vi "TCP.IP Server for Ripple Detection - edited for data 2.vi"() -> ()   [LabVIEW 2021]
doc: "Demonstrates how to set up a basic TCP connection, send data to the specified port once a connection has been established, and terminate the connection once the data has been sent. This VI is designed to stop if the TCP connection is terminated. The data sent in this example is an array of random numbers."
panel:
  out "error out":errorcluster
  in  "error in (no error)":errorcluster
  out "Numeric 3":dbl
  out "Waveform Graph 10":dynamicdata(graph)
  in  "loop 1":i32
  in  "Client Closed":string="The client VI closed the connection."
  in  "Stop":bool
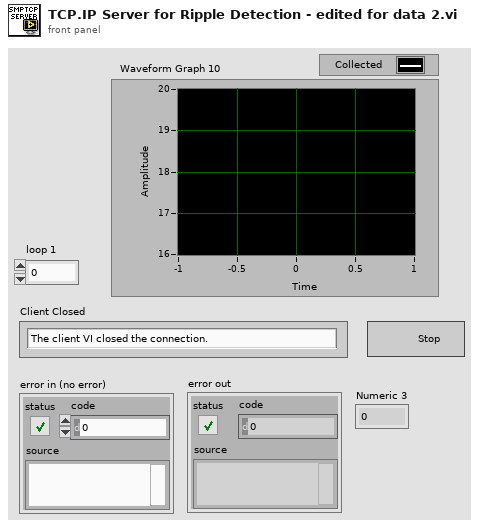
[diagram p1: front panel]
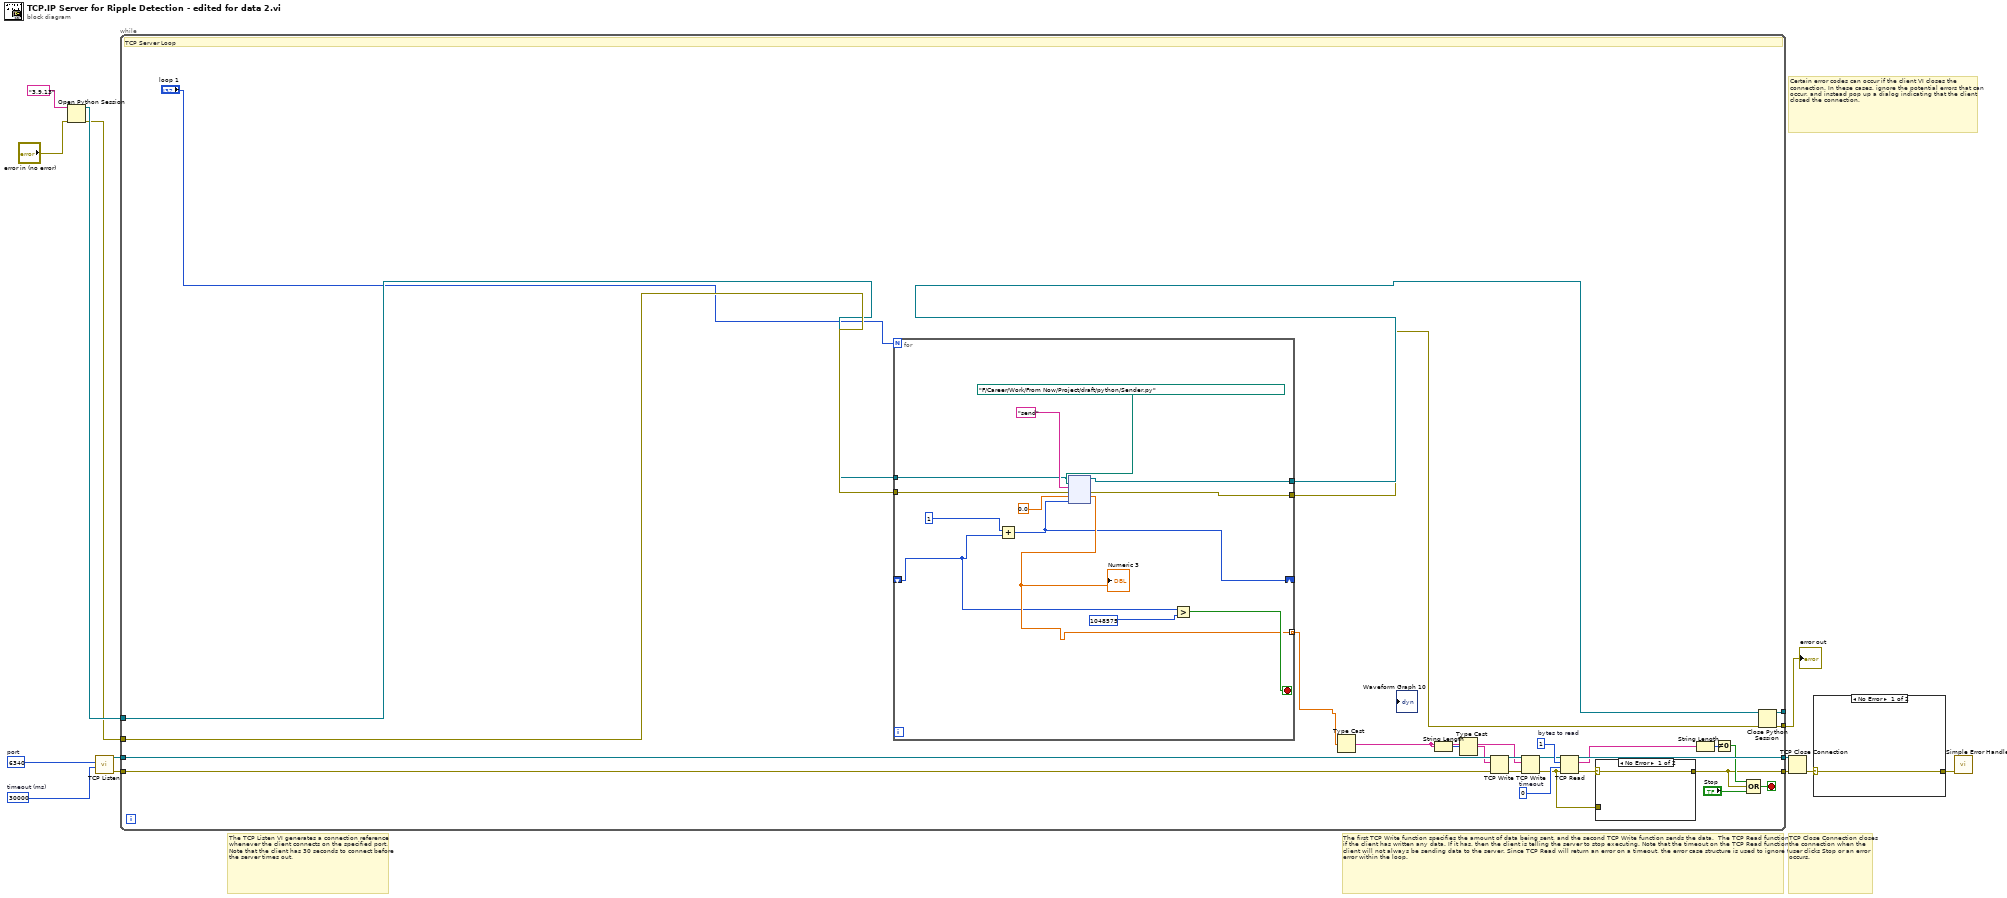
[diagram p0: block diagram]
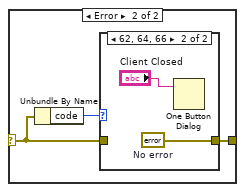
[diagram p2: hidden frame]
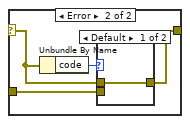
[diagram p4: hidden frame]
diagram:
  w8 = u16 6340  # port
  w9 = 30000  # timeout (ms)
  # "TCP Close Connection closes the connection when the user clicks Stop or an error occurs."
  # "The TCP Listen VI generates a connection reference whenever the client connects on the specified port. Note that the client has 30 seconds to connect before the server times out."
  # "Certain error codes can occur if the client VI closes the connection. In these cases, ignore the potential errors that can occur, and instead pop up a dialog indicating that the client closed the connection."
  # "The first TCP Write function specifies the amount of data being sent, and the second TCP Write function sends the data.  The TCP Read function checks to see if the client has written any data. If it has, then the client is telling the server to stop executing. Note that the timeout on the TCP Read function is '0', as the client will not always be sending data to the server. Since TCP Read will return an error on a timeout, the error case structure is used to ignore the timeout error within the loop."
  n1 = Open Python Session(python version="3.9.13" ("Python version"), 3:"error in (no error)") -> (session out=w6:refnum<k35>, error out=w5:errorcluster)  [unwired: 1 in]
  n2 = call <vilib>:"TCP Listen.vi"("timeout ms (wait forever: -1)"=w9, "port"=w8) -> ("error out"=w10:errorcluster, "connection ID"=w11:refnum<k5>)  [unwired: 5 in, 3 out]
  n3 = while {
    tunnel: [w23] -> w14
    tunnel: [w29] -> w15
    tunnel: w11 -> [w40]
    tunnel: w10 -> [w33]
    tunnel: w6 -> [w18]
    tunnel: w5 -> [w19]
    tunnel: [w21] -> w4
    tunnel: [w20] -> w3
    stop <- w34 stop-if-true
    w28 = 0  # timeout
    w31 = 1  # bytes to read
    # "TCP Server Loop"
    n4 = for {
      N: "loop 1" -> [_]
      tunnel: [w43] -> w16 mode=indexing
      tunnel: [w51] -> w21
      tunnel: [w50] -> w20
      tunnel: w18 -> [w49]
      tunnel: w19 -> [w48]
      shift-right: [w41] -> _
      shift-left: _ -> [w42]
      stop <- w47 stop-if-true
      n5 = Add(x=1, y=w42) -> (x+y=w41:i32)
      n6 = node(w49, path "F:/Career/Work/From Now/Project/draft/python/Sender.py" ("module path"), "send" ("function name"), w48, 0.0, w41) -> (w51:refnum<k35>, w50:errorcluster, w43:dbl)  [unwired: 1 in, 2 out]
      "Numeric 3" <- w43
      n7 = Greater?(x=w42, y=1048575) -> (0:w47:bool)
    }
    n8 = Type Cast(x=w16) -> (*(type *) &x=w35:string)  [unwired: 1 out]
    n9 = String Length(string=w35) -> (length=w37:i32)
    n10 = Type Cast(x=w37) -> (*(type *) &x=w36:string)  [unwired: 1 out]
    n11 = TCP Write(connection ID=w40, data in=w36, error in (no error)=w33) -> (connection ID out=w39:refnum<k5>, error out=w38:errorcluster)  [unwired: 2 out]
    n12 = TCP Write(connection ID=w39, data in=w35, error in (no error)=w38) -> (connection ID out=w30:refnum<k5>, error out=w22:errorcluster)  [unwired: 2 out]
    n13 = TCP Read(connection ID=w30, bytes to read=w31, error in (no error)=w22, 9:w28) -> (connection ID out=w29:refnum<k5>, data out=w26:string, error out=w24:errorcluster)  [unwired: 1 out]
    n14 = case shown="No Error" w24 {
      selector: w24 -> [w54 w57]
      tunnel: [w54 w55] -> w23
      tunnel: w22 -> [_ w56]
      frame No Error {
      }
      frame Error {
        n15 = Unbundle By Name(w57) -> ("code"=w58:i32)
        n16 = case shown="Default" w58 {
          tunnel: w57 -> [w59 _]
          tunnel: w56 -> [_ w60]
          tunnel: [w59 w60] -> w55
          frame Default {
          }
          frame 56 {
          }
        }
      }
    }
    n17 = String Length(string=w26) -> (length=w27:i32)
    n18 = Not Equal To 0?(x=w27) -> (x != 0?=w25:bool)
    n19 = Compound Arithmetic op=OR(w25, w23, "Stop") -> (w34:bool)
  }
  n20 = Close Python Session(session in=w4, error in=w3) -> (11:→"error out":errorcluster)
  n21 = TCP Close Connection(connection ID=w15, error in (no error)=w14) -> (error out=w13:errorcluster)  [unwired: 2 out]
  n22 = case shown="No Error" w13 {
    selector: w13 -> [w61 w63]
    tunnel: [w61 w62] -> w12
    frame No Error {
    }
    frame Error {
      n23 = Unbundle By Name(w63) -> ("code"=w64:i32)
      n24 = case shown="62, 64, 66" w64 {
        tunnel: w63 -> [w65 _]
        tunnel: [w65 w67] -> w62
        frame Default {
        }
        frame 62, 64, 66 {
          w67 = errorcluster {"status"=FALSE, "code"=0, "source"=""}  # No error
          n25 = One Button Dialog(message="Client Closed") -> ()  [unwired: 1 in, 1 out]
        }
      }
    }
  }
  n26 = call <vilib>:"Simple Error Handler.vi"("error in (no error)"=w12) -> ()  [unwired: 1 in, 8 out]
